vi "OAT Extract Orbit Timebase Data.vi"(5 "tach duty":i32=1, 7 "select output plot":u16(ring) items=["Orbit", "Timebase"], 8 "trigger pulse direction":u16(ring)=1 items=["positive going", "negative going"], 9 "duration":dbl format="%.2f", 10 "start points":dbl[](array[numeric]) format="%.2f", 11 "waveform data":waveform(dbl)) -> (0 "timebase plot":T1 {"timebase data" format="%.2f"; "timebase time" format="%.2f"}, 1 "tach points":cluster{"tach time":dbl[], "tach data":dbl[]} {"tach data" format="%.2f"; "tach time" format="%.2f"}, 2 "orbit data":dbl[](array[numeric]) format="%.2f", 3 "tach data":dbl[](array[numeric]) format="%.2f")   [LabVIEW 2017]
uses:
  <vilib>/Analysis/1siggen.llb/Ramp Pattern by Samples.vi
  <vilib>/Waveform/WDTOps.llb/WDT Get XY Value DBL.vi
  <vilib>/Waveform/WDTOps.llb/WDT Get Waveform Subset DBL.vi
  <vilib>/Analysis/NI_AALBase.lvlib
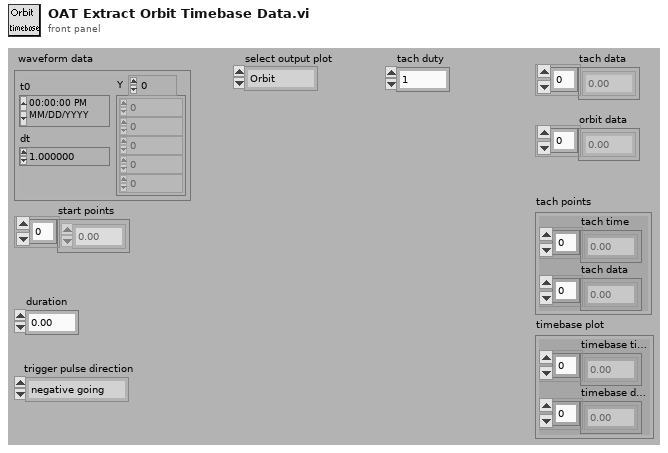
[diagram p1: front panel]
types:
  T1 = cluster{"timebase time":dbl[], "timebase data":dbl[]}
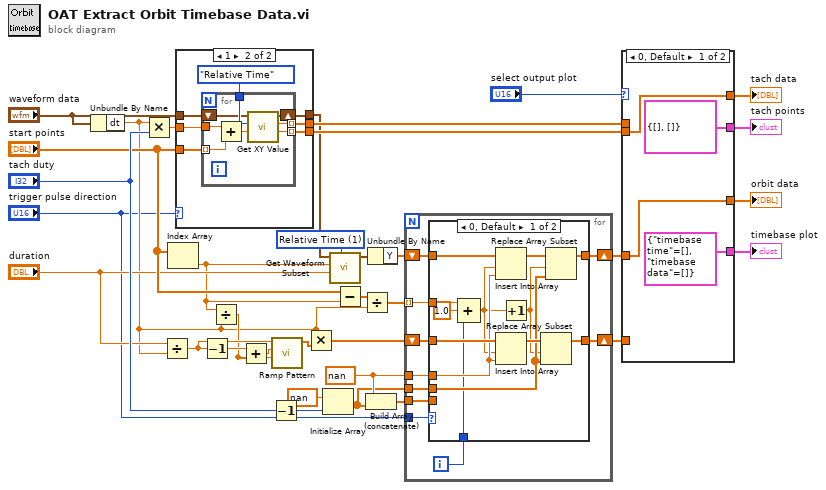
[diagram p0: block diagram]
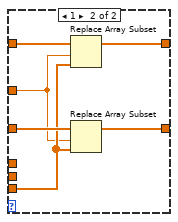
[diagram p2: hidden frame]
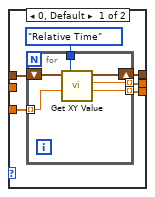
[diagram p3: hidden frame]
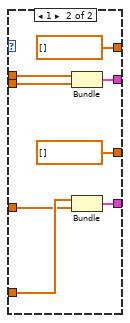
[diagram p4: hidden frame]
diagram:
  w2 = nan ("element")
  w27 = u16 1 items=["Index", "Relative Time"] ("Mode")
  n1 = Unbundle By Name("waveform data") -> ("dt"=w6:dbl)
  n2 = Multiply(x=w6, y="tach duty") -> (x*y=w28:dbl)
  n3 = Divide(x="duration", y=w6) -> (x/y=w14:dbl)
  n4 = Index Array(array="start points") -> (element=w15:dbl)  [unwired: 1 in]
  n5 = case shown="1" "trigger pulse direction" {
    tunnel: "waveform data" -> [w40 w50]
    tunnel: [w38 w52] -> w33
    tunnel: [w37 w51] -> w31
    tunnel: "start points" -> [w36 w49]
    tunnel: [w35 w48] -> w26
    tunnel: w28 -> [_ w47]
    frame 0, Default {
      n6 = for {
        shift-right: [w45] -> w35
        shift-left: w40 -> [w46]
        tunnel: w36 -> [w44] mode=indexing
        tunnel: [w43] -> w38 mode=indexing
        tunnel: [w42] -> w37 mode=indexing
        tunnel: enum16{"Index", "Relative Time"}."Relative Time" ("mode") -> [w41]
        n7 = call-poly <vilib>:"Get XY Value.vi"("Y position"=w44, "Y position format"=w41, "waveform in"=w46) -> ("Y value"=w43:dbl, "actual Y position"=w42:dbl, "waveform out"=w45:waveform(dbl))  [unwired: 4 in, 2 out]
      }
    }
    frame 1 {
      n8 = for {
        tunnel: enum16{"Index", "Relative Time"}."Relative Time" ("mode") -> [w61]
        shift-right: [w59] -> w48
        shift-left: w50 -> [w60]
        tunnel: w49 -> [w56] mode=indexing
        tunnel: [w58] -> w52 mode=indexing
        tunnel: [w57] -> w51 mode=indexing
        tunnel: w47 -> [w54]
        n9 = Add(x=w54, y=w56) -> (x+y=w55:dbl)
        n10 = call-poly <vilib>:"Get XY Value.vi"("Y position"=w55, "Y position format"=w61, "waveform in"=w60) -> ("Y value"=w58:dbl, "actual Y position"=w57:dbl, "waveform out"=w59:waveform(dbl))  [unwired: 4 in, 2 out]
      }
    }
  }
  n11 = Decrement(x=w14) -> (x-1=w13:dbl)
  n12 = Divide(x=w15, y=w6) -> (x/y=w12:dbl)
  n13 = Add(x=w13, y=w12) -> (x+y=w11:dbl)
  n14 = Decrement(x="tach duty") -> (x-1=w4:i32)
  n15 = call-poly <vilib>:"Ramp Pattern.vi"("start"=w12, "end"=w11, "samples"=w14) -> ("Ramp Pattern"=w10:dbl[])  [unwired: 7 in, 1 out]
  n16 = Multiply(x=w6, y=w10) -> (x*y=w7:dbl[])
  n17 = Initialize Array(nan ("element"), w4) -> (w1:dbl[])
  n18 = call-poly <vilib>:"Get Waveform Subset.vi"("start/duration format"=w27, "duration"="duration", "start samples/time"=w15, "waveform in"=w26) -> ("waveform out"=w23:waveform(dbl))  [unwired: 2 in, 3 out]
  n19 = Subtract(x="start points", y=w15) -> (x-y=w21:dbl[])
  n20 = Divide(x=w21, y=w6) -> (x/y=w19:dbl[])
  n21 = Build Array (concatenate)(w2, w1) -> (w3:dbl[])
  n22 = Unbundle By Name(w23) -> ("Y"=w20:dbl[])
  n23 = for {
    shift-right: [w70] -> w18
    shift-left: w20 -> [w71]
    tunnel: w19 -> [w68] mode=indexing
    tunnel: w3 -> [w65]
    shift-right: [w67] -> w9
    shift-left: w7 -> [w69]
    tunnel: "trigger pulse direction" -> [w66]
    tunnel: w2 -> [w64]
    tunnel: w1 -> [w63]
    i -> [w62]
    n24 = case shown="0, Default" w66 {
      tunnel: w71 -> [w84 w90]
      tunnel: [w80 w89] -> w70
      tunnel: w69 -> [w83 w88]
      tunnel: w65 -> [_ w87]
      tunnel: w68 -> [w75 w86]
      tunnel: [w78 w85] -> w67
      tunnel: w64 -> [w82 _]
      tunnel: w63 -> [w77 _]
      tunnel: w62 -> [w74 _]
      frame 0, Default {
        n25 = Compound Arithmetic op=ADD(w75, 1.0 ("value"), w74) -> (w72:dbl)
        n26 = Insert Into Array(array=w84, index=w72, new element=w82) -> (w81:dbl[])
        n27 = Insert Into Array(array=w83, index=w72, new element=w82) -> (w79:dbl[])
        n28 = Increment(x=w72) -> (x+1=w76:dbl)
        n29 = Replace Array Subset(array=w79, new element=w77, index=w76) -> (w78:dbl[])
        n30 = Replace Array Subset(array=w81, new element=w77, index=w76) -> (w80:dbl[])
      }
      frame 1 {
        n31 = Replace Array Subset(array=w90, new element=w87, index=w86) -> (w89:dbl[])
        n32 = Replace Array Subset(array=w88, new element=w87, index=w86) -> (w85:dbl[])
      }
    }
  }
  n33 = case shown="0, Default" "select output plot" {
    tunnel: w33 -> [w94 w101]
    tunnel: [w94 dbl[] []] -> w32
    tunnel: w31 -> [_ w102]
    tunnel: [cluster{dbl[], dbl[]} {[], []} w100] -> w30
    tunnel: w18 -> [w92 w96]
    tunnel: [w92 dbl[] [] ("Y")] -> w17
    tunnel: w9 -> [_ w97]
    tunnel: [T1 {"timebase time"=[], "timebase data"=[]} ("timebase line") w95] -> w8
    frame 0, Default {
    }
    frame 1 {
      n34 = Bundle(w102, w101) -> (w100:cluster{dbl[], dbl[]})  [unwired: 1 in]
      n35 = Bundle(w97, "Y"=w96) -> (w95:cluster{dbl[], "Y":dbl[]})  [unwired: 1 in]
    }
  }
  "tach points" <- w30
  "tach data" <- w32
  "orbit data" <- w17
  "timebase plot" <- w8
